vi "test.vi"() -> ()   [LabVIEW 2016]
panel:
  out "VI Name":string
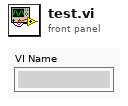
[diagram p1: front panel]
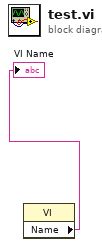
[diagram p0: block diagram]
diagram:
  n1 = property class="VI"() -> ("Name"=→"VI Name":string)  [unwired: 2 in, 2 out]
